vi "建立全局变量.vi"() -> ()   [LabVIEW 2010]
panel:
  in  "操作者姓名":string
  out "报警":bool
  in  "温度":dbl
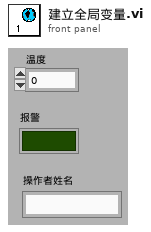
[diagram p1: front panel]
diagram:
